vi "Z900_navX_Internal_Get.vi"(8 "error in (no error)":errorcluster, 11 "navX Device":T1={"Interface"={"Protocol"=enum."SERIAL", "Update Rate (4Hz-100Hz)"=4, "navX Open TypeDef"=variant}, "Notify Packet"=refnum, "Loop VI Refnum"=refnum, "Ready to Close Occurrence Refnum"=refnum} {"Interface"."Update Rate (4Hz-100Hz)" min=4 max=60 step=1}) -> (0 "error out":errorcluster, 1 "Connected":bool, 2 "Registry":u8[](array[numeric]), 3 "navX Device":T1={"Interface"={"Protocol"=enum."SERIAL", "Update Rate (4Hz-100Hz)"=4, "navX Open TypeDef"=variant}, "Notify Packet"=refnum, "Loop VI Refnum"=refnum, "Ready to Close Occurrence Refnum"=refnum} {"Interface"."Update Rate (4Hz-100Hz)" min=4 max=60 step=1})   [LabVIEW 2016, in "navX Library v2.lvlib"]
doc: "This VI returns the current values from the navX device registy. This VI is rarely need to be called by a user."
uses:
  navX Library v2.lvlib
  TypeDefs/Z900_navX_DeviceTypeDef.ctl
  TypeDefs/Z900_navX_ProtocolTypeDef.ctl
  TypeDefs/Z900_navX_NotifyPacketTypeDef.ctl
  TypeDefs/Z900_navX_ActionTypeDef.ctl
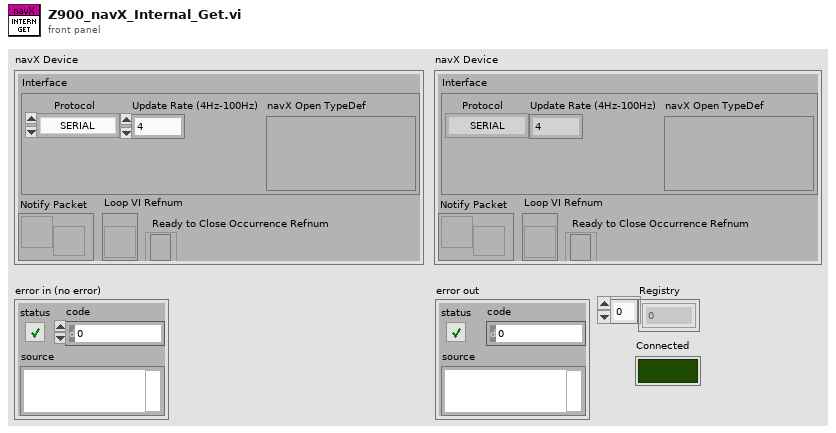
[diagram p1: front panel]
types:
  T1 = typedef "navX Library v2.lvlib/Z900_navX_DeviceTypeDef.ctl" = cluster{"Interface":cluster{"Protocol":T2, "Update Rate (4Hz-100Hz)":u8, "navX Open TypeDef":variant}, "Notify Packet":refnum<notifier>, "Loop VI Refnum":refnum<vi>, "Ready to Close Occurrence Refnum":refnum<k4>}
  T2 = typedef "navX Library v2.lvlib/Z900_navX_ProtocolTypeDef.ctl" = enum16{"SERIAL", "I2C", "SPI"}
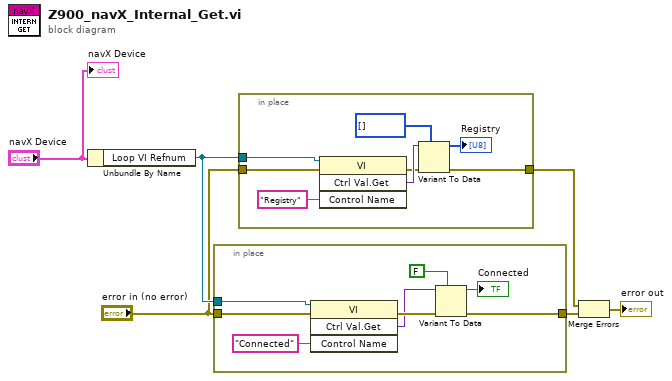
[diagram p0: block diagram]
diagram:
  n1 = Unbundle By Name("navX Device") -> ("Loop VI Refnum"=w2:refnum<vi>)
  n2 = in-place {
    in-place-border: [w9] -> w3
    in-place-border: w2 -> [w8]
    in-place-border: "error in (no error)" -> [w7]
    n3 = invoke class="VI" method="Ctrl Val.Get"(reference=w8, error in=w7, "Control Name"="Connected") -> (error out=w14:errorcluster, "Get Control Value Variant"=w13:variant)  [unwired: 1 in, 2 out]
    n4 = Variant To Data(error in=w14, type=FALSE, Variant=w13) -> (data=→"Connected":bool, error out=w9:errorcluster)
  }
  n5 = in-place {
    in-place-border: [w17] -> w5
    in-place-border: w2 -> [w16]
    in-place-border: "error in (no error)" -> [w15]
    n6 = invoke class="VI" method="Ctrl Val.Get"(reference=w16, error in=w15, "Control Name"="Registry") -> (error out=w18:errorcluster, "Get Control Value Variant"=w21:variant)  [unwired: 1 in, 2 out]
    n7 = Variant To Data(error in=w18, type=u8[] [], Variant=w21) -> (data=→"Registry":u8[], error out=w17:errorcluster)
  }
  n8 = Merge Errors(w5, w3) -> (→"error out":errorcluster)
  "navX Device" <- "navX Device"
